vi "bool_edge_on.vi"(11 "Input":bool) -> (3 "On Edge":bool)   [LabVIEW 2020]
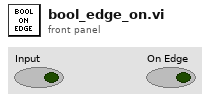
[diagram p1: front panel]
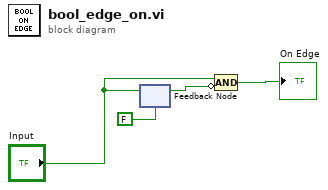
[diagram p0: block diagram]
diagram:
  n1 = feedback #1(FALSE ("Robot Enabled")) -> (w2:bool)
  n2 = feedback-in #1("Input") -> ()
  n3 = Compound Arithmetic op=AND("Input", invert w2) -> (→"On Edge":bool)
